vi "Chess.vi"() -> ()   [LabVIEW 2019]
uses:
  #typedef_ProgramStates.ctl
  #typedef_SpecialMoves.ctl
  #typedef_Color.ctl
panel:
  out "Instruction":string
  in  "Exit":bool
  in  "Start":bool
  out "?":u16[][](array[ring])
  # "8"
  # "7"
  # "6"
  # "5"
  # "4"
  # "3"
  # "2"
  # "1"
  # "c"
  # "d"
  # "e"
  # "f"
  # "g"
  # "h"
  # "a"
  # "b"
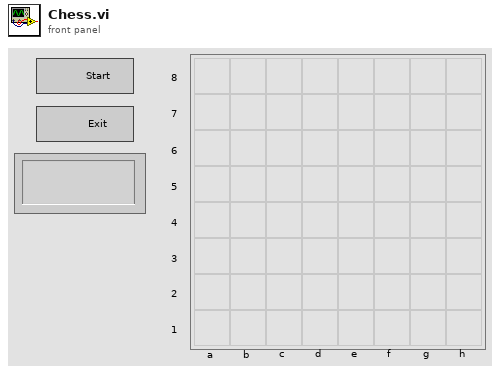
[diagram p1: front panel]
types:
  T1 = typedef "#typedef_ProgramStates.ctl" = enum16{"Init", "Clicking on Piece", "Clicking on Square", "Checking Movement", "Checking King  ", "Checking if Mate", "End"}
  T2 = typedef "#typedef_SpecialMoves.ctl" = enum16{"None", "Last Square", "Beat in the Passage", "Short Castle", "Long Castle"}
  T3 = typedef "#typedef_Color.ctl" = enum16{"White", "Black"}
  T4 = typedef "#typedef_DataBase.ctl" = cluster{"Squares type":T5[][], "Turn":T3, "Move from":i32[], "Move to":i32[], "Instruction":string, "Board":T8[][], "Special Moves":T2}
  T5 = typedef "#typedef_SquareType.ctl" = cluster{"Square Color":T3, "Position":i32[], "Piece":T6}
  T6 = typedef "#typedef_Piece.ctl" = cluster{"Type":T7, "Color":T3, "Moved?":bool}
  T7 = typedef "#typedef_PieceType.ctl" = enum16{"None", "Pawn", "Knight", "Bishop", "Rook", "Queen", "King"}
  T8 = typedef "#typedef_SquareLook.ctl" = u16
  T9 = typedef "LVPositionTypeDef.ctl" = cluster{"Left":i32, "Top":i32}
  T10 = typedef "LVBoundsTypeDef.ctl" = cluster{"Width":u32, "Height":u32}
  T11 = typedef "LVPoint32TypeDef.ctl" = cluster{"Horizontal":i32, "Vertical":i32}
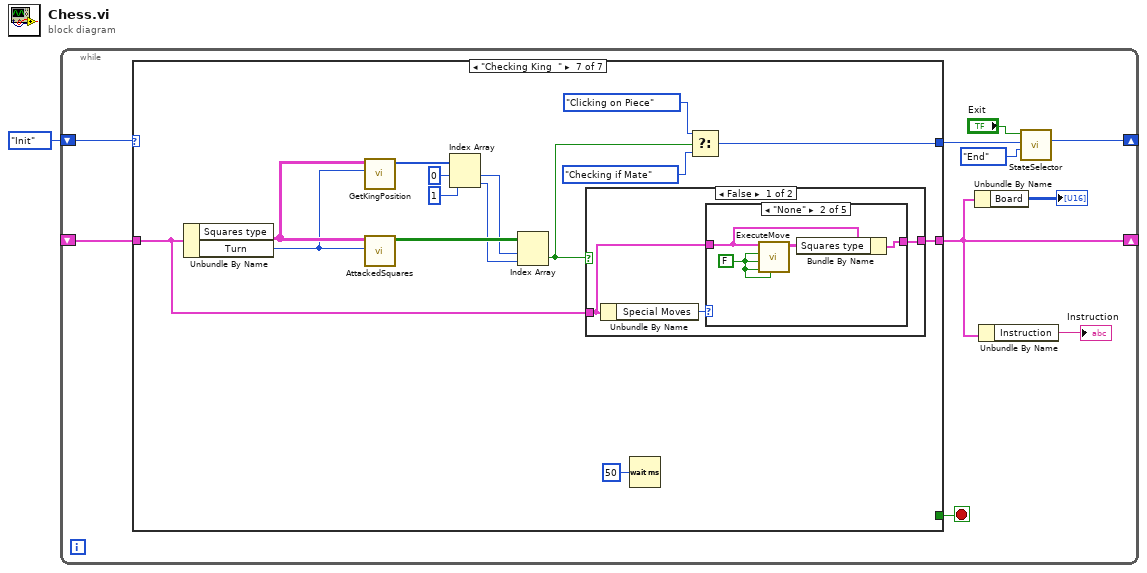
[diagram p0: block diagram]
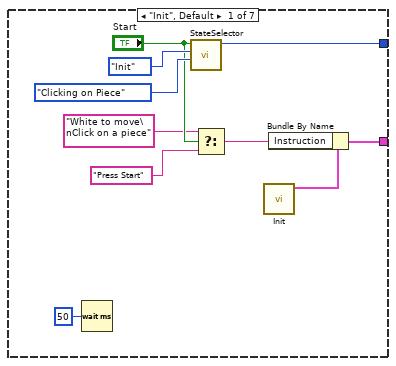
[diagram p2: hidden frame]
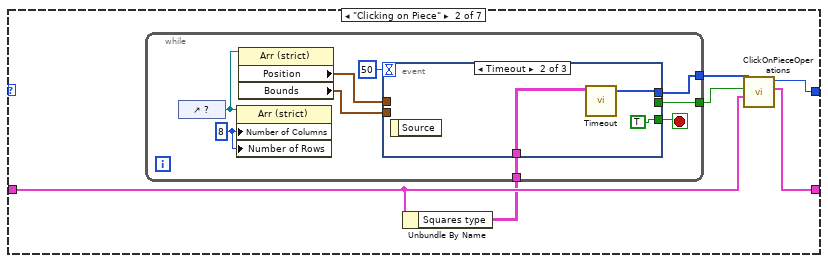
[diagram p3: hidden frame]
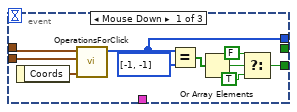
[diagram p4: hidden frame]
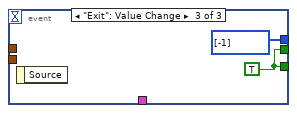
[diagram p5: hidden frame]
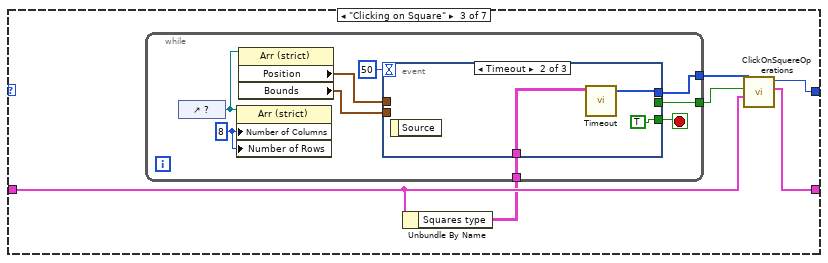
[diagram p6: hidden frame]
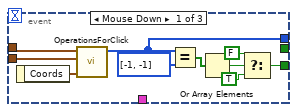
[diagram p7: hidden frame]
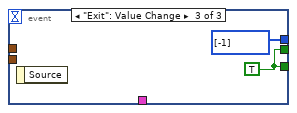
[diagram p8: hidden frame]
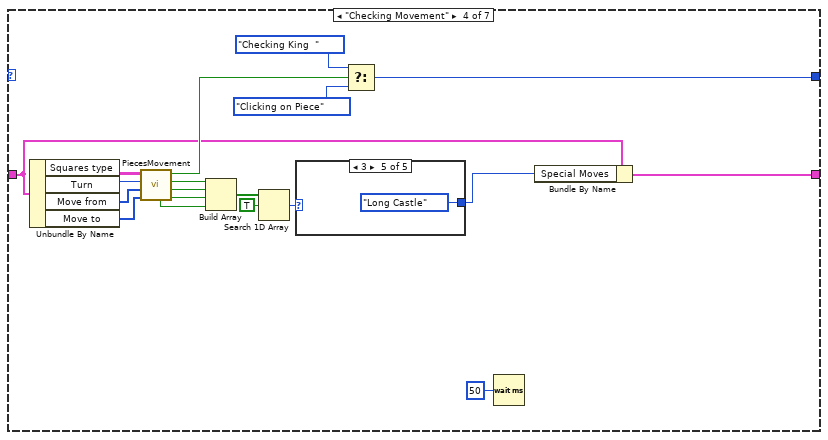
[diagram p9: hidden frame]
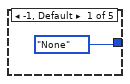
[diagram p10: hidden frame]
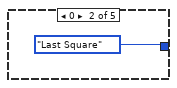
[diagram p11: hidden frame]
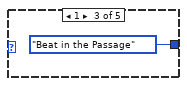
[diagram p12: hidden frame]
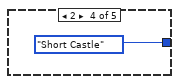
[diagram p13: hidden frame]
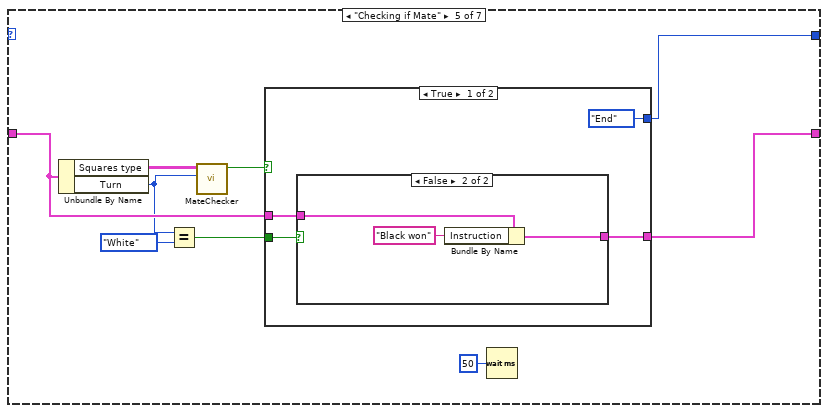
[diagram p14: hidden frame]
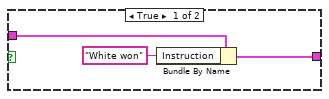
[diagram p15: hidden frame]
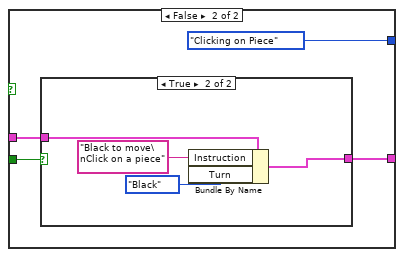
[diagram p16: hidden frame]
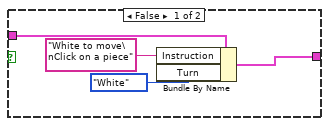
[diagram p17: hidden frame]
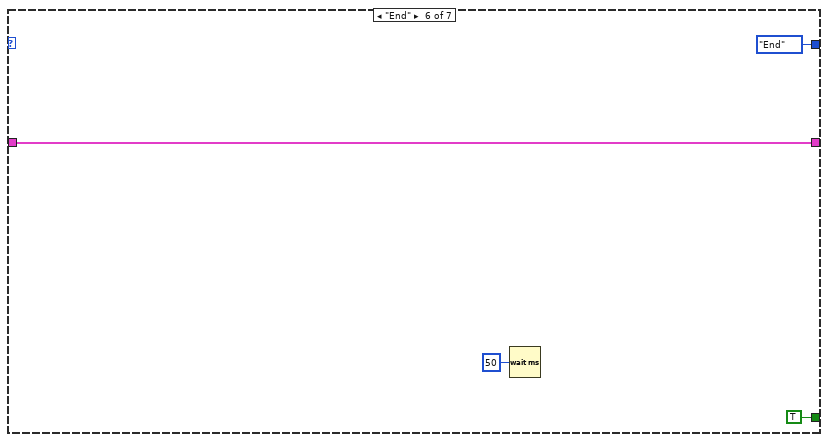
[diagram p18: hidden frame]
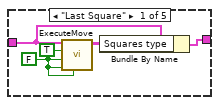
[diagram p19: hidden frame]
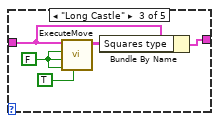
[diagram p20: hidden frame]
diagram:
  n1 = while {
    shift-right: [w3] -> _
    shift-left: _ -> [w6]
    shift-right: [w8] -> _
    shift-left: #typedef_ProgramStates."Init" -> [w11]
    stop <- w7 stop-if-true
    n2 = case shown="\"Checking King  \"" w11 {
      tunnel: [w16 w26 w56 w94 w107 w139 w142] -> w3
      tunnel: [w20 w24 w54 w90 w106 #typedef_ProgramStates."End" ("Output State") w145] -> w9
      tunnel: [_ _ _ _ _ TRUE _] -> w7
      tunnel: w6 -> [_ w23 w53 w87 w111 w139 w143]
      frame "Init", Default {
        n3 = Wait (ms)(milliseconds to wait=u32 50) -> ()  [unwired: 1 out]
        n4 = call "StateSelector.vi"("Conditional State"=#typedef_ProgramStates."Clicking on Piece", "Default State"=#typedef_ProgramStates."Init", "Action Button"="Start") -> ("Output State"=w20:T1)  [unwired: 8 in]
        n5 = Select(t="White to move\nClick on a piece", s="Start", f="Press Start") -> (s? t:f=w14:string)
        n6 = call "Init.vi"() -> ("Initialized DataBase"=w17:T4)  [unwired: 11 in]
        n7 = Bundle By Name(cluster=w17, "Instruction"=w14) -> (w16:T4)
      }
      frame "Clicking on Piece" {
        n8 = Unbundle By Name(w23) -> ("Squares type"=w22:T5[][])
        n9 = while {
          tunnel: [w35] -> w27
          tunnel: [w33] -> w25
          tunnel: w22 -> [w28]
          stop <- w34 stop-if-true
          w31 = u32 8 ("Number of Columns")
          n10 = control-ref of="?"() -> (w32:refnum<vi>)
          n11 = property on="Property Node" class="Arr (strict)"(reference=w32, "Number of Columns"=w31, "Number of Rows"=w31) -> ()  [unwired: 1 in, 2 out]
          n12 = property on="Property Node" class="Arr (strict)"(reference=w32) -> ("Position"=w30:T9, "Bounds"=w29:T10)  [unwired: 1 in, 2 out]
          n13 = event shown="[1] Timeout" {
            selector: _ -> [_ _ _]
            dyn-events: _ -> [_ _ _]
            timeout: 50 -> [_ _ _]
            tunnel: [w37 w48 i32[] [-1] ("Clicked Position")] -> w35
            tunnel: w30 -> [w44 _ _]
            tunnel: w29 -> [w45 _ _]
            tunnel: [w38 TRUE ("t") w50] -> w34
            tunnel: [_ _ w50] -> w33
            tunnel: w28 -> [_ w47 _]
            event Mouse Down {
              n14 = event-data() -> ("Coords"=w46:T11)  [unwired: 1 in]
              n15 = call "OperationsForClick.vi"("Input Coords"=w46, "Input Bounds"=w45, "Input Position"=w44) -> ("Clicked Position"=w37:i32[])  [unwired: 8 in]
              n16 = Equal?(x=w37, y=i32[] [-1, -1]) -> (x = y?=w42:bool[])
              n17 = Or Array Elements(Boolean array=w42) -> (logical OR=w41:bool)
              n18 = Select(t=FALSE, s=w41, f=TRUE) -> (s? t:f=w38:bool)
            }
            event Timeout {
              n19 = event-data() -> ()  [unwired: 1 in, 1 out]
              n20 = call "Timeout.vi"("Squares type"=w47) -> ("Clicked Position"=w48:i32[])  [unwired: 10 in]
            }
            event "Exit": Value Change {
              w50 = TRUE
              n21 = event-data() -> ()  [unwired: 1 in, 1 out]
            }
          }
        }
        n22 = call "ClickOnPieceOperations.vi"("Input DataBase"=w23, "Off Board?"=w25, "Clicked Position"=w27) -> ("Output DataBase"=w26:T4, "Output State"=w24:T1)  [unwired: 7 in]
      }
      frame "Clicking on Square" {
        n23 = Unbundle By Name(w53) -> ("Squares type"=w52:T5[][])
        n24 = while {
          tunnel: [w65] -> w57
          tunnel: [w63] -> w55
          tunnel: w52 -> [w58]
          stop <- w64 stop-if-true
          w61 = u32 8 ("Number of Columns")
          n25 = control-ref of="?"() -> (w62:refnum<vi>)
          n26 = property on="Property Node" class="Arr (strict)"(reference=w62, "Number of Columns"=w61, "Number of Rows"=w61) -> ()  [unwired: 1 in, 2 out]
          n27 = property on="Property Node" class="Arr (strict)"(reference=w62) -> ("Position"=w60:T9, "Bounds"=w59:T10)  [unwired: 1 in, 2 out]
          n28 = event shown="[1] Timeout" {
            selector: _ -> [_ _ _]
            dyn-events: _ -> [_ _ _]
            timeout: 50 -> [_ _ _]
            tunnel: [w67 w78 i32[] [-1] ("Clicked Position")] -> w65
            tunnel: w60 -> [w74 _ _]
            tunnel: w59 -> [w75 _ _]
            tunnel: [w68 TRUE ("t") w80] -> w64
            tunnel: [_ _ w80] -> w63
            tunnel: w58 -> [_ w77 _]
            event Mouse Down {
              n29 = event-data() -> ("Coords"=w76:T11)  [unwired: 1 in]
              n30 = call "OperationsForClick.vi"("Input Coords"=w76, "Input Bounds"=w75, "Input Position"=w74) -> ("Clicked Position"=w67:i32[])  [unwired: 8 in]
              n31 = Equal?(x=w67, y=i32[] [-1, -1]) -> (x = y?=w72:bool[])
              n32 = Or Array Elements(Boolean array=w72) -> (logical OR=w71:bool)
              n33 = Select(t=FALSE, s=w71, f=TRUE) -> (s? t:f=w68:bool)
            }
            event Timeout {
              n34 = event-data() -> ()  [unwired: 1 in, 1 out]
              n35 = call "Timeout.vi"("Squares type"=w77) -> ("Clicked Position"=w78:i32[])  [unwired: 10 in]
            }
            event "Exit": Value Change {
              w80 = TRUE
              n36 = event-data() -> ()  [unwired: 1 in, 1 out]
            }
          }
        }
        n37 = call "ClickOnSquereOperations.vi"("Input DataBase"=w53, "Off Board?"=w55, "Clicked Position"=w57) -> ("Output DataBase"=w56:T4, "Output State"=w54:T1)  [unwired: 7 in]
      }
      frame "Checking Movement" {
        n38 = Unbundle By Name(w87) -> ("Squares type"=w86:T5[][], "Turn"=w85:T3, "Move from"=w84:i32[], "Move to"=w83:i32[])
        n39 = call "PiecesMovement.vi"("Move to"=w83, "Move from"=w84, "Turn"=w85, "Input Squares"=w86) -> ("Short Castle?"=w98:bool, "Beat in the Passage?"=w99:bool, "Last Square?"=w100:bool, "Possible Move?"=w93:bool, "Long Castle?"=w89:bool)  [unwired: 2 in, 1 out]
        n40 = Build Array(w100, w99, w98, w89) -> (w97:bool[])
        n41 = Search 1D Array(1D array=w97, element=TRUE) -> (index of element=w95:i32)  [unwired: 1 in]
        n42 = case shown="3" w95 {
          tunnel: [#typedef_SpecialMoves."None" #typedef_SpecialMoves."Last Square" #typedef_SpecialMoves."Beat in the Passage" #typedef_SpecialMoves."Short Castle" #typedef_SpecialMoves."Long Castle"] -> w88
          frame -1, Default {
          }
          frame 0 {
          }
          frame 1 {
          }
          frame 2 {
          }
          frame 3 {
          }
        }
        n43 = Select(t=#typedef_ProgramStates."Checking King  " ("Conditional State"), s=w93, f=#typedef_ProgramStates."Clicking on Piece") -> (s? t:f=w90:T1)
        n44 = Wait (ms)(milliseconds to wait=u32 50) -> ()  [unwired: 1 out]
        n45 = Bundle By Name(cluster=w87, "Special Moves"=w88) -> (w94:T4)
      }
      frame "Checking if Mate" {
        n46 = Unbundle By Name(w111) -> ("Squares type"=w113:T5[][], "Turn"=w110:T3)
        n47 = Equal?(x=w110, y=#typedef_Color."White") -> (x = y?=w108:bool)
        n48 = call "MateChecker.vi"("Turn"=w110, "Input Squares"=w113) -> ("Checkmate?"=w112:bool)  [unwired: 9 in]
        n49 = case shown="True" w112 {
          tunnel: w111 -> [w117 w127]
          tunnel: w108 -> [w118 w128]
          tunnel: [w116 w126] -> w107
          tunnel: [#typedef_ProgramStates."End" ("f") #typedef_ProgramStates."Clicking on Piece" ("f")] -> w106
          frame True {
            n50 = case shown="False" w118 {
              tunnel: w117 -> [w121 w124]
              tunnel: [w119 w122] -> w116
              frame True {
                n51 = Bundle By Name(cluster=w121, "Instruction"="White won") -> (w119:T4)
              }
              frame False {
                n52 = Bundle By Name(cluster=w124, "Instruction"="Black won") -> (w122:T4)
              }
            }
          }
          frame False {
            n53 = case shown="True" w128 {
              tunnel: w127 -> [w132 w136]
              tunnel: [w130 w134] -> w126
              frame False {
                n54 = Bundle By Name(cluster=w132, "Instruction"="White to move\nClick on a piece", "Turn"=#typedef_Color."White") -> (w130:T4)
              }
              frame True {
                n55 = Bundle By Name(cluster=w136, "Instruction"="Black to move\nClick on a piece", "Turn"=#typedef_Color."Black") -> (w134:T4)
              }
            }
          }
        }
        n56 = Wait (ms)(milliseconds to wait=u32 50) -> ()  [unwired: 1 out]
      }
      frame "End" {
        n57 = Wait (ms)(milliseconds to wait=u32 50) -> ()  [unwired: 1 out]
      }
      frame "Checking King  " {
        n58 = Unbundle By Name(w143) -> ("Squares type"=w155:T5[][], "Turn"=w154:T3)
        n59 = call "GetKingPosition.vi"("Color"=w154, "Input Squares"=w155) -> ("Position"=w153:i32[])  [unwired: 9 in]
        n60 = call "AttackedSquares.vi"("Turn"=w154, "Input Squares"=w155) -> ("Attacked Squares"=w150:bool[][])  [unwired: 9 in]
        n61 = Index Array(array=w153, index #1=0 ("index"), index #2=1 ("index")) -> (element #1=w149:i32, element #2=w148:i32)
        n62 = Index Array(array=w150, index (row)=w149, index (col)=w148) -> (element=w144:bool)
        n63 = case shown="False" w144 {
          tunnel: w143 -> [w157 w183]
          tunnel: [w156 w183] -> w142
          frame False {
            n64 = Unbundle By Name(w157) -> ("Special Moves"=w158:T2)
            n65 = case shown="\"None\"" w158 {
              tunnel: w157 -> [w162 w166 w171 w176 w181]
              tunnel: [w160 w164 w169 w174 w179] -> w156
              frame "Last Square" {
                w163 = FALSE ("Last Square?")
                n66 = call "ExecuteMove.vi"("Long Castle?"=w163, "Small Castle?"=w163, "In the Passage?"=w163, "Last Square?"=TRUE, "Input DataBase"=w162) -> ("Output Squares"=w161:T5[][])  [unwired: 6 in]
                n67 = Bundle By Name(cluster=w162, "Squares type"=w161) -> (w160:T4)
              }
              frame "None" {
                w167 = FALSE ("Last Square?")
                n68 = call "ExecuteMove.vi"("Long Castle?"=w167, "Small Castle?"=w167, "In the Passage?"=w167, "Last Square?"=w167, "Input DataBase"=w166) -> ("Output Squares"=w165:T5[][])  [unwired: 6 in]
                n69 = Bundle By Name(cluster=w166, "Squares type"=w165) -> (w164:T4)
              }
              frame "Long Castle" {
                w172 = FALSE ("Last Square?")
                n70 = call "ExecuteMove.vi"("Long Castle?"=TRUE ("Big Castle?"), "Small Castle?"=w172, "In the Passage?"=w172, "Last Square?"=w172, "Input DataBase"=w171) -> ("Output Squares"=w170:T5[][])  [unwired: 6 in]
                n71 = Bundle By Name(cluster=w171, "Squares type"=w170) -> (w169:T4)
              }
              frame "Short Castle" {
                w177 = FALSE ("Last Square?")
                n72 = call "ExecuteMove.vi"("Long Castle?"=w177, "Small Castle?"=TRUE, "In the Passage?"=w177, "Last Square?"=w177, "Input DataBase"=w176) -> ("Output Squares"=w175:T5[][])  [unwired: 6 in]
                n73 = Bundle By Name(cluster=w176, "Squares type"=w175) -> (w174:T4)
              }
              frame "Beat in the Passage" {
                w182 = FALSE ("Last Square?")
                n74 = call "ExecuteMove.vi"("Long Castle?"=w182, "Small Castle?"=w182, "In the Passage?"=TRUE, "Last Square?"=w182, "Input DataBase"=w181) -> ("Output Squares"=w180:T5[][])  [unwired: 6 in]
                n75 = Bundle By Name(cluster=w181, "Squares type"=w180) -> (w179:T4)
              }
            }
          }
          frame True {
          }
        }
        n76 = Wait (ms)(milliseconds to wait=u32 50) -> ()  [unwired: 1 out]
        n77 = Select(t=#typedef_ProgramStates."Clicking on Piece" ("Conditional State"), s=w144, f=#typedef_ProgramStates."Checking if Mate") -> (s? t:f=w145:T1)
      }
    }
    n78 = Unbundle By Name(w3) -> ("Board"=→"?":T8[][])
    n79 = Unbundle By Name(w3) -> ("Instruction"=→"Instruction":string)
    n80 = call "StateSelector.vi"("Conditional State"=#typedef_ProgramStates."End", "Default State"=w9, "Action Button"="Exit") -> ("Output State"=w8:T1)  [unwired: 8 in]
  }
